vi "UMLEditor_CreateCursors.vi"(8 "error in (no error)":errorcluster) -> (0 "error out":errorcluster, 3 "Array":refnum<k1>[](array[refnum]))   [LabVIEW 2020]
uses:
  <resource>/Framework/Providers/Open_GDS/UML/UMLEditor/UMLEditor_Cursortype.ctl
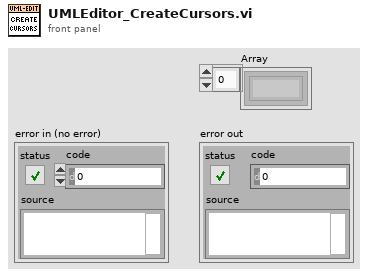
[diagram p1: front panel]
types:
  T1 = typedef "UMLEditor_Cursortype.ctl" = enum16{"Arrow", "Move", "Finger", "Wait", "NS", "WE", "NESW", "NWSE"}
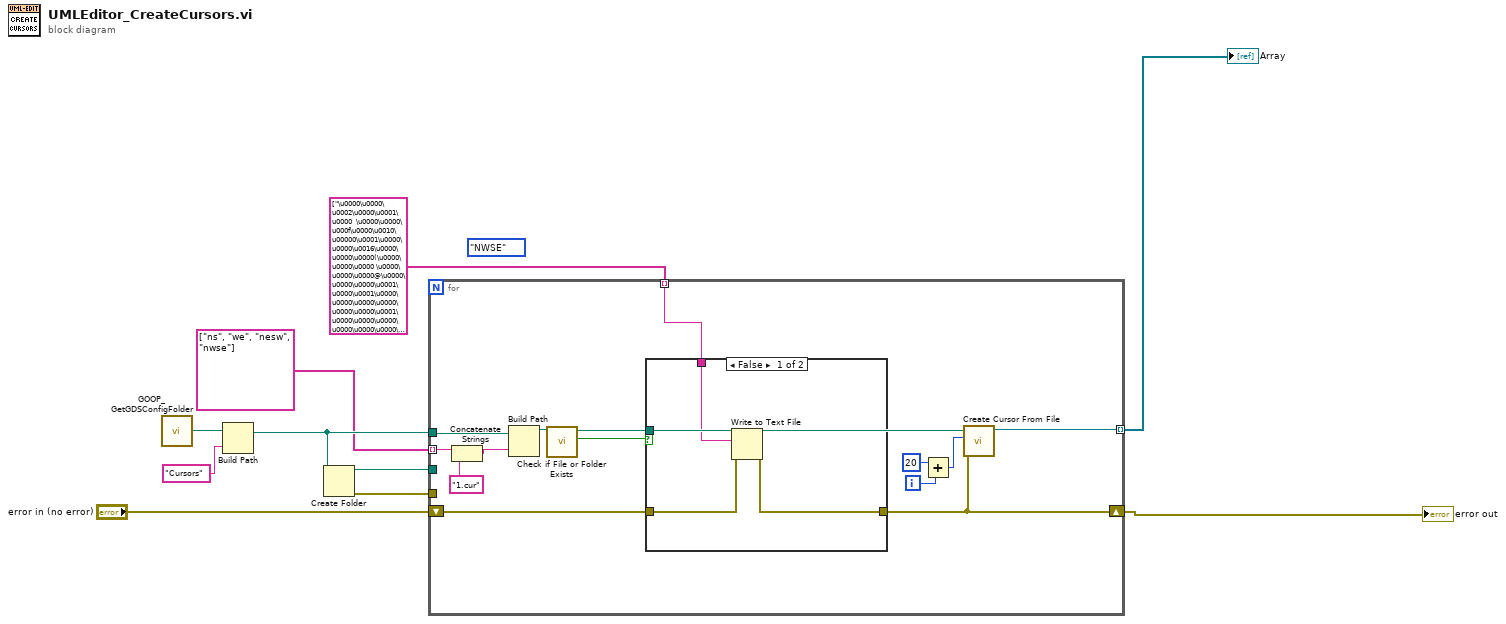
[diagram p0: block diagram]
diagram:
  (unwired) UMLEditor_Cursortype."NWSE" ("CursorType")
  n1 = call <resource>:"GOOP_GetGDSConfigFolder.vi"() -> ("GDSFolderPath"=w5:path)
  n2 = Build Path(base path=w5, name or relative path="Cursors") -> (appended path=w8:path)
  n3 = Create Folder(path (use dialog)=w8) -> (created path=w9:path, error out=w10:errorcluster)  [unwired: 2 in, 1 out]
  n4 = for {
    tunnel: w8 -> [w24]
    tunnel: string[] ["ns", "we", "nesw", "nwse"] -> [w20] mode=indexing
    shift-right: [w11] -> w3
    shift-left: "error in (no error)" -> [w14]
    tunnel: [w21] -> w4 mode=indexing
    tunnel: string[] ["\u0000\u0000\u0002\u0000\u0001\u0000  \u0000\u0000\u000f\u0000\u0010\u00000\u0001\u0000\u0000\u0016\u0000\u0000\u0000(\u0000\u0000\u0000 \u0000\u0000\u0000@\u0000\u0000\u0000\u0001\u0000\u0001\u0000\u0000\u0000\u0000\u0000\u0000\u0001\u0000\u0000\u0000\u0000\u0000\u0000\u0000\u0000\u0000\u0000\u0000\u0000\u0000\u0000\u0000\u0000\u0000\u0000\u0000\u0000\u0000\u0000ÿÿÿ\u0000\u0000\u0000\u0000\u0000\u0000\u0000\u0000\u0000\u0000\u0000\u0000\u0000\u0000\u0000\u0000\u0000\u0000\u0000\u0000\u0000\u0000\u0001\u0000\u0000\u0000\u0002€\u0000\u0000\u0004@\u0000\u0000\b \u0000\u0000\u0010\u0010\u0000\u0000\u001eð\u0000\u0000\u0002€\u0000\u0000\u0002€\u0000\u0000\u0002€\u0000\u0000\u0002€\u0000\u0000\u0002€\u0000\u0000\u0002€\u0000\u0000\u0002€\u0000\u0000\u0002€\u0000\u0000\u001eð\u0000\u0000\u0010\u0010\u0000\u0000\b \u0000\u0000\u0004@\u0000\u0000\u0002€\u0000\u0000\u0001\u0000\u0000\u0000\u0000\u0000\u0000\u0000\u0000\u0000\u0000\u0000\u0000\u0000\u0000\u0000\u0000\u0000\u0000\u0000\u0000\u0000\u0000\u0000\u0000\u0000\u0000\u0000\u0000\u0000\u0000ÿÿÿÿÿÿÿÿÿÿÿÿÿÿÿÿÿÿÿÿÿþÿÿÿüÿÿø?ÿÿð\u001fÿÿà\u000fÿÿà\u000fÿÿüÿÿüÿÿüÿÿüÿÿüÿÿüÿÿüÿÿüÿÿà\u000fÿÿà\u000fÿÿð\u001fÿÿø?ÿÿüÿÿþÿÿÿÿÿÿÿÿÿÿÿÿÿÿÿÿÿÿÿÿÿÿÿÿÿÿÿÿÿÿ", "\u0000\u0000\u0002\u0000\u0001\u0000  \u0000\u0000\u0010\u0000\u0010\u00000\u0001\u0000\u0000\u0016\u0000\u0000\u0000(\u0000\u0000\u0000 \u0000\u0000\u0000@\u0000\u0000\u0000\u0001\u0000\u0001\u0000\u0000\u0000\u0000\u0000\u0000\u0001\u0000\u0000\u0000\u0000\u0000\u0000\u0000\u0000\u0000\u0000\u0000\u0000\u0000\u0000\u0000\u0000\u0000\u0000\u0000\u0000\u0000\u0000ÿÿÿ\u0000\u0000\u0000\u0000\u0000\u0000\u0000\u0000\u0000\u0000\u0000\u0000\u0000\u0000\u0000\u0000\u0000\u0000\u0000\u0000\u0000\u0000\u0000\u0000\u0000\u0000\u0000\u0000\u0000\u0000\u0000\u0000\u0000\u0000\u0000\u0000\u0000\u0000\u0000\u0000\u0000\u0000\u0000\u0000\u0000\u00000\u0006\u0000\u0000P\u0005\u0000\u0000\u0004\u0001\u001fü@\u0002\u0000\u0000 \u0001\u001fü@\u0000\u0004\u0000P\u0005\u0000\u00000\u0006\u0000\u0000\u0000\u0000\u0000\u0000\u0000\u0000\u0000\u0000\u0000\u0000\u0000\u0000\u0000\u0000\u0000\u0000\u0000\u0000\u0000\u0000\u0000\u0000\u0000\u0000\u0000\u0000\u0000\u0000\u0000\u0000\u0000\u0000\u0000\u0000\u0000\u0000\u0000\u0000\u0000\u0000\u0000\u0000\u0000\u0000\u0000\u0000\u0000ÿÿÿÿÿÿÿÿÿÿÿÿÿÿÿÿÿÿÿÿÿÿÿÿÿÿÿÿÿÿÿÿÿÿÿÿÿÿÿÿÿÿÿÿÿÏùÿÿøÿÿ\u000føþ\u0000\u0000?ü\u0000\u0000\u001fþ\u0000\u0000?ÿ\u000føÿøÿÿÏùÿÿÿÿÿÿÿÿÿÿÿÿÿÿÿÿÿÿÿÿÿÿÿÿÿÿÿÿÿÿÿÿÿÿÿÿÿÿÿÿÿÿÿÿÿÿÿÿÿ", "\u0000\u0000\u0002\u0000\u0001\u0000  \u0000\u0000\u0010\u0000\u0010\u00000\u0001\u0000\u0000\u0016\u0000\u0000\u0000(\u0000\u0000\u0000 \u0000\u0000\u0000@\u0000\u0000\u0000\u0001\u0000\u0001\u0000\u0000\u0000\u0000\u0000\u0000\u0001\u0000\u0000\u0000\u0000\u0000\u0000\u0000\u0000\u0000\u0000\u0000\u0000\u0000\u0000\u0000\u0000\u0000\u0000\u0000\u0000\u0000\u0000ÿÿÿ\u0000\u0000\u0000\u0000\u0000\u0000\u0000\u0000\u0000\u0000\u0000\u0000\u0000\u0000\u0000\u0000\u0000\u0000\u0000\u0000\u0000\u0000\u0000\u0000\u0000\u0000\u0000\u0000\u0000\u0000\u0000\u0000\u0000\u0000\u0000\u0000\u0000A\u0000\u0000\u0000B\u0000\u0000\u0000D\u0000\u0000\u0000J\u0000\u0000\u0000U\u0000\u0000\u0000b\u0000\u0000\u0001@\u0000\u0000\u0000£\u0000\u0000\u0000U\u0000\u0000\u0000)\u0000\u0000\u0000\u0011\u0000\u0000\u0000!\u0000\u0000\u0000A\u0000\u0000\u0000\u0000\u0000\u0000\u0000\u0000\u0000\u0000\u0000\u0000\u0000\u0000\u0000\u0000\u0000\u0000\u0000\u0000\u0000\u0000\u0000\u0000\u0000\u0000\u0000\u0000\u0000\u0000\u0000\u0000\u0000\u0000\u0000\u0000\u0000\u0000\u0000\u0000ÿÿÿÿÿÿÿÿÿÿÿÿÿÿÿÿÿÿÿÿÿÿÿÿÿÿÿÿÿÿÿÿÿÿÿÿÿÿÿÿÿÿÿÿÿÿÿÿÿÿÿÿÿþ?ÿÿÿ\u001cÿÿÿÿÿÿÀÿÿÿàÿÿÿÀÿÿÿÿÿÿÿÿÿÿÿÿÿÿÿÿÿÿÿÿÿÿÿÿÿÿÿÿÿÿÿÿÿÿÿÿÿÿÿÿÿÿÿ", "\u0000\u0000\u0002\u0000\u0001\u0000  \u0000\u0000\u0010\u0000\u0010\u00000\u0001\u0000\u0000\u0016\u0000\u0000\u0000(\u0000\u0000\u0000 \u0000\u0000\u0000@\u0000\u0000\u0000\u0001\u0000\u0001\u0000\u0000\u0000\u0000\u0000\u0000\u0001\u0000\u0000\u0000\u0000\u0000\u0000\u0000\u0000\u0000\u0000\u0000\u0000\u0000\u0000\u0000\u0000\u0000\u0000\u0000\u0000\u0000\u0000ÿÿÿ\u0000\u0000\u0000\u0000\u0000\u0000\u0000\u0000\u0000\u0000\u0000\u0000\u0000\u0000\u0000\u0000\u0000\u0000\u0000\u0000\u0000\u0000\u0000\u0000\u0000\u0000\u0000\u0000\u0000\u0000\u0000\u0000\u0000\u0000\u0000\u0000\u0000\u0000A\u0000\u0000\u0000!\u0000\u0000\u0000\u0011\u0000\u0000\u0000)\u0000\u0000\u0000U\u0000\u0000\u0000£\u0000\u0000\u0001@\u0000\u0000b\u0000\u0000U\u0000\u0000\u0000J\u0000\u0000\u0000D\u0000\u0000\u0000B\u0000\u0000\u0000A\u0000\u0000\u0000\u0000\u0000\u0000\u0000\u0000\u0000\u0000\u0000\u0000\u0000\u0000\u0000\u0000\u0000\u0000\u0000\u0000\u0000\u0000\u0000\u0000\u0000\u0000\u0000\u0000\u0000\u0000\u0000\u0000\u0000\u0000\u0000\u0000\u0000\u0000\u0000\u0000\u0000ÿÿÿÿÿÿÿÿÿÿÿÿÿÿÿÿÿÿÿÿÿÿÿÿÿÿÿÿÿÿÿÿÿÿÿÿÿÿÿÿÀÿÿÿàÿÿÿÀÿÿÿÿÿÿ\u001cÿÿþ?ÿÿÿÿÿÿÿÿÿÿÿÿÿÿÿÿÿÿÿÿÿÿÿÿÿÿÿÿÿÿÿÿÿÿÿÿÿÿÿÿÿÿÿÿÿÿÿÿÿÿÿÿÿÿÿÿÿ"] -> [w12] mode=indexing
    tunnel: w9 -> [_]
    tunnel: w10 -> [_]
    i -> [w23]
    n5 = Concatenate Strings(w20, "1.cur" ("string")) -> (w18:string)
    n6 = Build Path(base path=w24, name or relative path=w18) -> (appended path=w16:path)
    n7 = call <vilib>:"Check if File or Folder Exists.vi"("path"=w16) -> ("file or folder exists?"=w15:bool, "dup path"=w13:path)  [unwired: 8 in, 1 out]
    n8 = case shown="False" w15 {
      tunnel: w14 -> [w28 w29]
      tunnel: [w27 w29] -> w11
      tunnel: w13 -> [w26 _]
      tunnel: w12 -> [w25 _]
      frame False {
        n9 = Write to Text File(file (use dialog)=w26, text=w25, error in=w28) -> (error out=w27:errorcluster)  [unwired: 1 in, 2 out]
      }
      frame True {
      }
    }
    n10 = Add(x=i16 20 ("cursor resource ID"), y=w23) -> (x+y=w17:i32)
    n11 = call <vilib>:"Create Cursor From File.vi"("error in (no error)"=w11, "cursor resource ID"=w17, "cursor file"=w13) -> ("cursor ID"=w21:refnum<k1>)  [unwired: 1 in, 7 out]
  }
  "Array" <- w4
  "error out" <- w3
